vi "Read SlotTime(ms).vi"(8 "error in (no error)":errorcluster, 11 "FrameSlot_Root in":refnum<class "FrameSlot_Root.lvclass">) -> (0 "error out":errorcluster, 2 "SlotTime(ms)":dbl, 3 "FrameSlot_Root out":refnum<class "FrameSlot_Root.lvclass">)   [LabVIEW 2018, in "FrameSlot_Root.lvclass"]
uses:
  FrameSlot_Root.lvclass
  FrameSlot_Root.lvclass/FrameSlot_Root.ctl
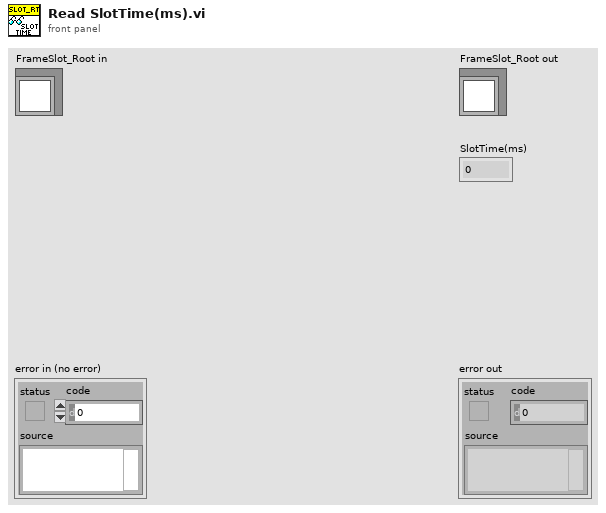
[diagram p1: front panel]
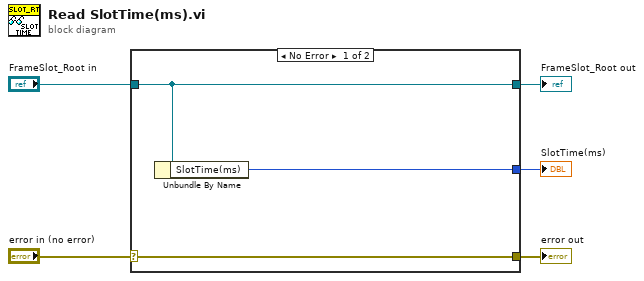
[diagram p0: block diagram]
diagram:
  n1 = case shown="No Error" "error in (no error)" {
    selector: "error in (no error)" -> [w8 w9]
    tunnel: [w8 w9] -> w4
    tunnel: [w7 w10] -> w2
    tunnel: "FrameSlot_Root in" -> [w7 w10]
    tunnel: [w6 _] -> w1
    frame No Error {
      n2 = Unbundle By Name(w7) -> ("SlotTime(ms)"=w6:u32)
    }
    frame Error {
    }
  }
  "error out" <- w4
  "FrameSlot_Root out" <- w2
  "SlotTime(ms)" <- w1
